vi "Generate Pump State Event.vi"(8 "error in (no error)":errorcluster, 10 "Pump State":T1, 11 "Pump in":refnum<class "Pump.lvclass">) -> (0 "error out":errorcluster, 3 "Pump out":refnum<class "Pump.lvclass">)   [LabVIEW 2014, in "Pump.lvclass"]
uses:
  Pump.lvclass
  Pump State - cluster.ctl
  Pump.lvclass/Pump.ctl
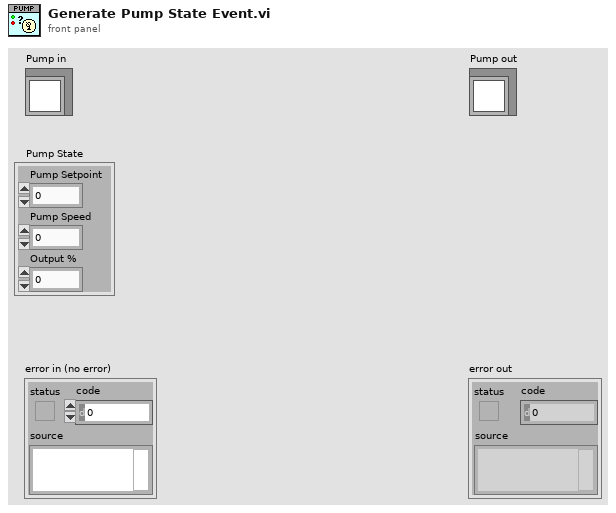
[diagram p1: front panel]
types:
  T1 = typedef "Pump.lvclass/Pump State - cluster.ctl" = cluster{"Pump Setpoint":dbl, "Pump Speed":dbl, "Output %":dbl}
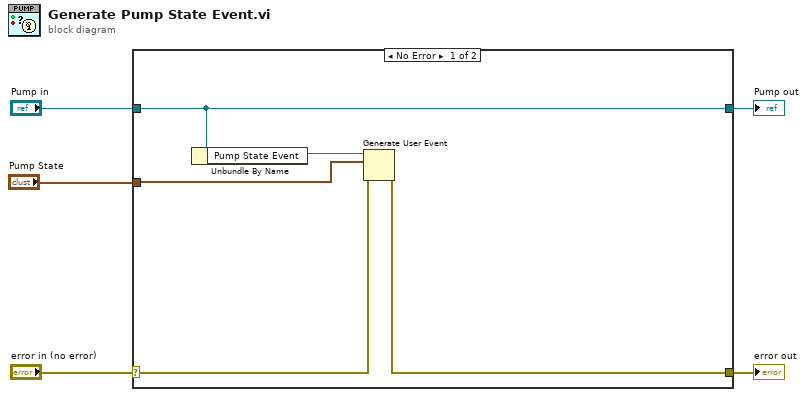
[diagram p0: block diagram]
diagram:
  n1 = case shown="No Error" "error in (no error)" {
    selector: "error in (no error)" -> [w7 w12]
    tunnel: [w6 w12] -> w4
    tunnel: [w10 w11] -> w2
    tunnel: "Pump in" -> [w10 w11]
    tunnel: "Pump State" -> [w8 _]
    frame No Error {
      n2 = Unbundle By Name(w10) -> ("Pump State Event"=w9:refnum<user-event>)
      n3 = Generate User Event(user event=w9, event data cluster=w8, error in=w7) -> (error out=w6:errorcluster)  [unwired: 1 in, 1 out]
    }
    frame Error {
    }
  }
  "error out" <- w4
  "Pump out" <- w2
